vi "FPGA-7842R-Control V1.vi"(0 "Waveform Data":T4, 2 "Action":T5=enum."Exit", 5 "Laser Controls":T1 {"405 Power (0-5V)" min=0.0 max=5.0}, 7 "Manual Controls":T3={"Galvo 1 Position (I16)"=-280, "Galvo 2 Position (I16)"=-280, "X Axis Voltage (I16)"=0, "Y Axis Voltage (I16)"=0, "Z Axis Voltage (I16)"=0, "Res Mirror Amp (I16)"=0, "Res Mirror Mute"=FALSE}, 9 "Image Acquisition Parameters":T2={"Scan Type"=enum."Sample Scanning", "Scan Mode"=enum."XY", "Fast Axis Frequency (Hz)"=100.0, "Image Format"=128, "Line Accumulations"=1, "Frames Per Capture"=1, "Frames Accumulations"=1, "Image Dimension (um)"=[], "Number of Z Steps"=1, "Z Steps Size (um)"=1.0, "Pixel Size (nm)"=[]} {"Z Steps Size (um)" min=0.0; "Number of Z Steps" min=1; "Frames Accumulations" min=1; "Frames Per Capture" min=1; "Line Accumulations" min=1; "Image Format" items=["64 x 64"=64, "128 x 128"=128, "256 x 256"=256, "512 x 512"=512, "1024 x 1024"=1024, "2048 x 2048"=2048]}, 11 "Initialize":bool, 12 "Unused Axis Offset (I16)":i16) -> (15 "Initalized":bool)   [LabVIEW 2016]
uses:
  <vilib>/rvi/interface/nirviOpenFPGA/nirviOpenFPGA.xnode
  <vilib>/rvi/interface/nirviMethod/nirviMethod.xnode
  <vilib>/rvi/interface/nirviReadWriteControl/nirviReadWriteControl.xnode
  <vilib>/rvi/interface/nirviCloseFPGA/nirviCloseFPGA.xnode
  FPGA Bitfiles/MainSTEDFPGAProj_FPGATarget_WaveformandLaser_XaHwHstXqlY.lvbitx
  FPGA Target VIs/FPGA-7841R/Waveform and Laser Controls V6.vi
  <vilib>/FPGAPlugInAG/PCIe-7841R/niLvFpga_Open_PCIe-7841R.vi
  FPGA Target VIs/FPGA-7841R/Waveform Scan Parameters.ctl
  NiFpgaLv.dll
  <vilib>/Utility/error.llb/Error Cluster From Error Code.vi
  <vilib>/rvi/errors/niLvFpgaAdjustHostInterfaceError.vi
  <vilib>/FPGAPlugInAG/PCIe-7841R/niLvFpga_Run_PCIe-7841R.vi
  <vilib>/FPGAPlugInAG/PCIe-7841R/niLvFpga_Close_PCIe-7841R.vi
  Waveform Data.ctl
  FPGA-7842R-Reference.ctl
  Manual Controls V2.ctl
  Type Defs/Image Acquisition Parameters.ctl
  Laser Controls.ctl
panel:
  in  "Laser State 02":bool[](array[boolean])=[FALSE, FALSE, TRUE, FALSE, FALSE, FALSE, FALSE, FALSE]
  in  "Laser State 01":bool[](array[boolean])=[FALSE, TRUE, FALSE, FALSE, FALSE, FALSE, FALSE, FALSE]
  in  "Two Color Line by Line":bool
  in  "Laser On Time (Ticks)":u8=25
  in  "Laser Delay (Ticks)":u8=25
  # "XY"
  # "Z"
  # "Length"
  # "Height"
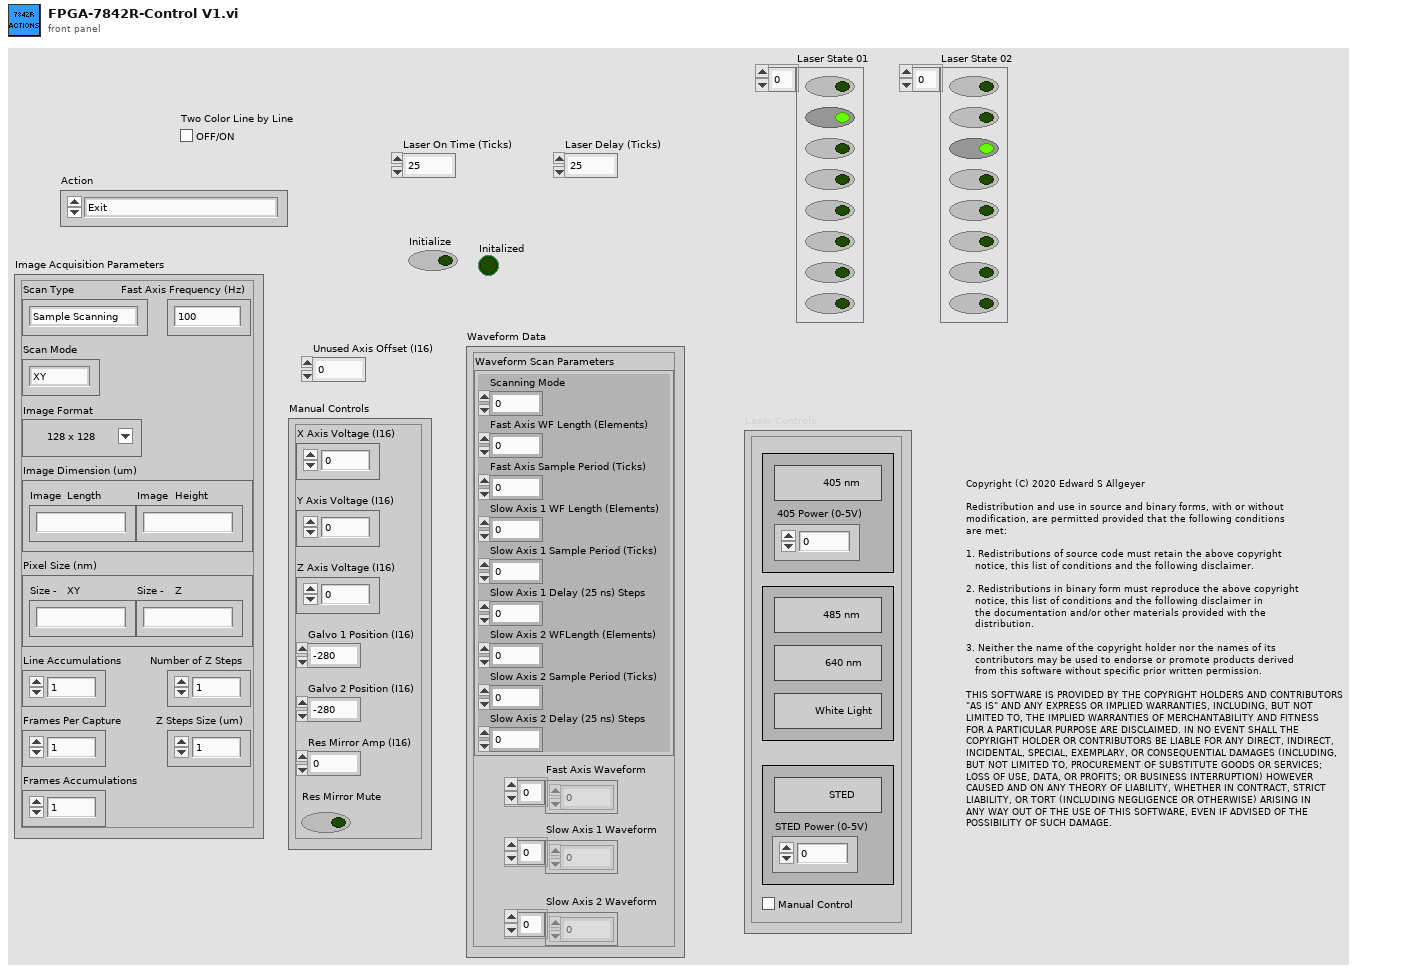
[diagram p1: front panel]
types:
  T1 = typedef "Laser Controls.ctl" = cluster{"STED Power (0-5V)":dbl, "STED":bool, "640 nm":bool, "485 nm":bool, "Manual Control":bool, "White Light":bool, "405 nm":bool, "405 Power (0-5V)":dbl}
  T2 = typedef "Image Acquisition Parameters.ctl" = cluster{"Scan Type":enum16{"Sample Scanning", "Beam Scanning"}, "Scan Mode":enum16{"XY", "XZ", "YZ", "XYZ"}, "Fast Axis Frequency (Hz)":dbl, "Image Format":u16, "Line Accumulations":u16, "Frames Per Capture":u16, "Frames Accumulations":u16, "Image Dimension (um)":dbl[], "Number of Z Steps":u8, "Z Steps Size (um)":dbl, "Pixel Size (nm)":dbl[]}
  T3 = typedef "Manual Controls V2.ctl" = cluster{"Galvo 1 Position (I16)":i16, "Galvo 2 Position (I16)":i16, "X Axis Voltage (I16)":i16, "Y Axis Voltage (I16)":i16, "Z Axis Voltage (I16)":i16, "Res Mirror Amp (I16)":i16, "Res Mirror Mute":bool}
  T4 = typedef "Waveform Data.ctl" = cluster{"Waveform Scan Parameters":cluster{"Scanning Mode":u8, "Fast Axis WF Length (Elements)":i32, "Fast Axis Sample Period (Ticks)":u32, "Slow Axis 1 WF Length (Elements)":i32, "Slow Axis 1 Sample Period (Ticks)":u32, "Slow Axis 1 Delay (25 ns) Steps":i32, "Slow Axis 2 WFLength (Elements)":i32, "Slow Axis 2 Sample Period (Ticks)":u32, "Slow Axis 2 Delay (25 ns) Steps":i32}, "Fast Axis Waveform":dbl[], "Slow Axis 1 Waveform":dbl[], "Slow Axis 2 Waveform":dbl[]}
  T5 = typedef "FPGA-7842R-Reference.ctl" = enum16{"Stage Control", "Laser Control", "Unused Axis I16", "Exit", "Set Res Mirror", "Set Galvo", "Default", "Close FPGA", "Stop Waveforms", "Start Waveforms", "Initialize"}
  T6 = cluster{"Scanning Mode":u8, "Fast Axis WF Length (Elements)":i32, "Fast Axis Sample Period (Ticks)":u32, "Slow Axis 1 WF Length (Elements)":i32, "Slow Axis 1 Sample Period (Ticks)":u32, "Slow Axis 1 Delay (25 ns) Steps":i32, "Slow Axis 2 WFLength (Elements)":i32, "Slow Axis 2 Sample Period (Ticks)":u32, "Slow Axis 2 Delay (25 ns) Steps":i32}
  T7 = cluster{"Res Mirror Amp (I16)":i16, "Res Mirror Mute":bool}
  T8 = typedef "Scan Parameters.ctl" = cluster{"Fast_Ax_Amp_V":dbl, "Fast_Ax_Off_V":dbl, "Slow_Ax_Amp_V":dbl, "Slow_Ax_Off_V ":dbl, "Slow_Ax_Max_V_VperS":dbl, "Slow_Ax1_Del25ns":i32, "Slow_Ax2_Del25ns":i32, "Stage_X_Off_V":dbl, "Stage_Y_Off_V":dbl, "Stage_Z_Off_V":dbl, "Galvo1_Off_V":dbl, "Galvo2_Off_V":dbl, "Last_Scan_Mode":enum16{"XY", "XZ", "YZ", "XYZ"}, "Current_Scan_Mode":enum16{"XY", "XZ", "YZ", "XYZ"}, "Fly_Back_Lines":u16, "Linear_Ramp_End":u32, "Z_Step_I16":i16, "Z_Start_I16":i16, "Laser_States _U32":u32, "590_Voltage_I16":i16, "775_AOM_Volt_I16":i16, "Blanking OFF":bool, "Unused_Axis_I16":i16}
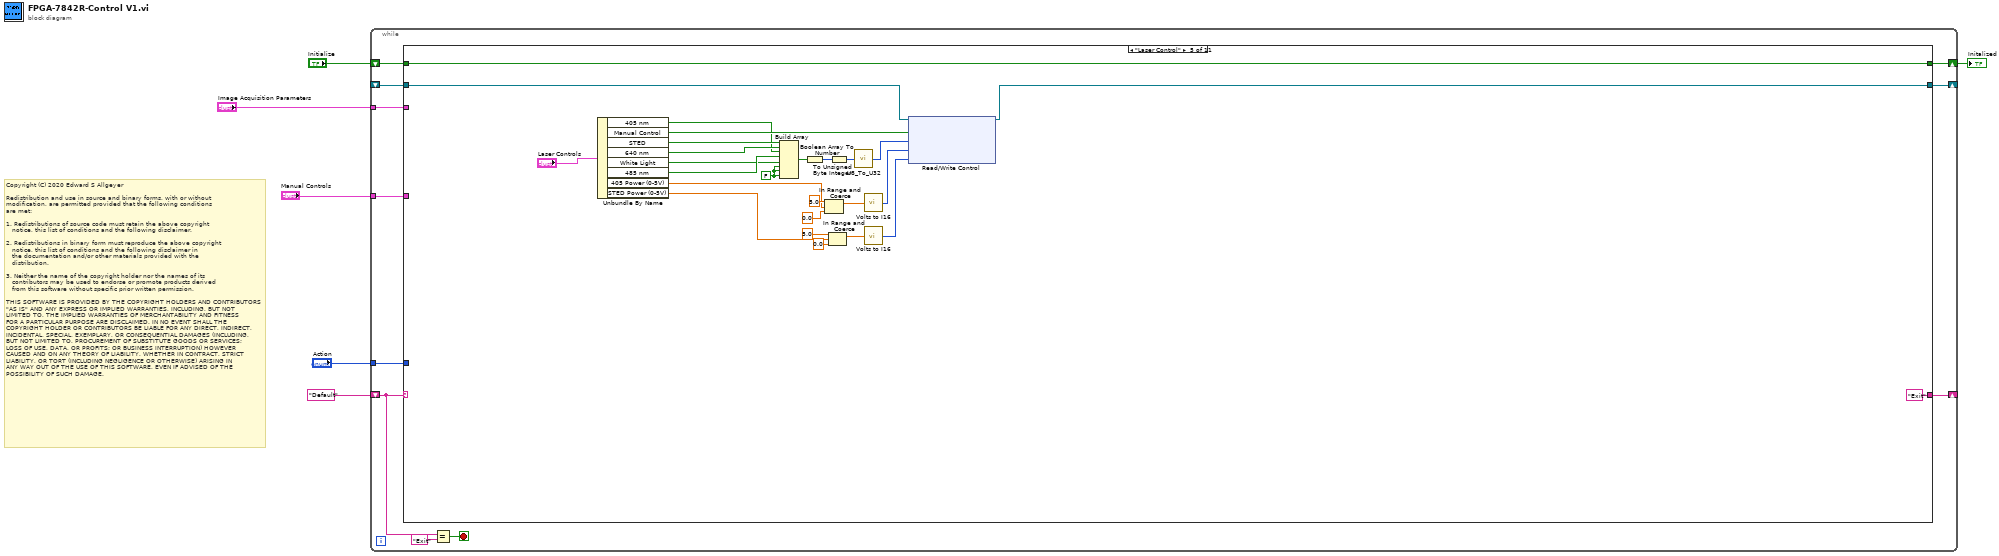
[diagram p0: block diagram]
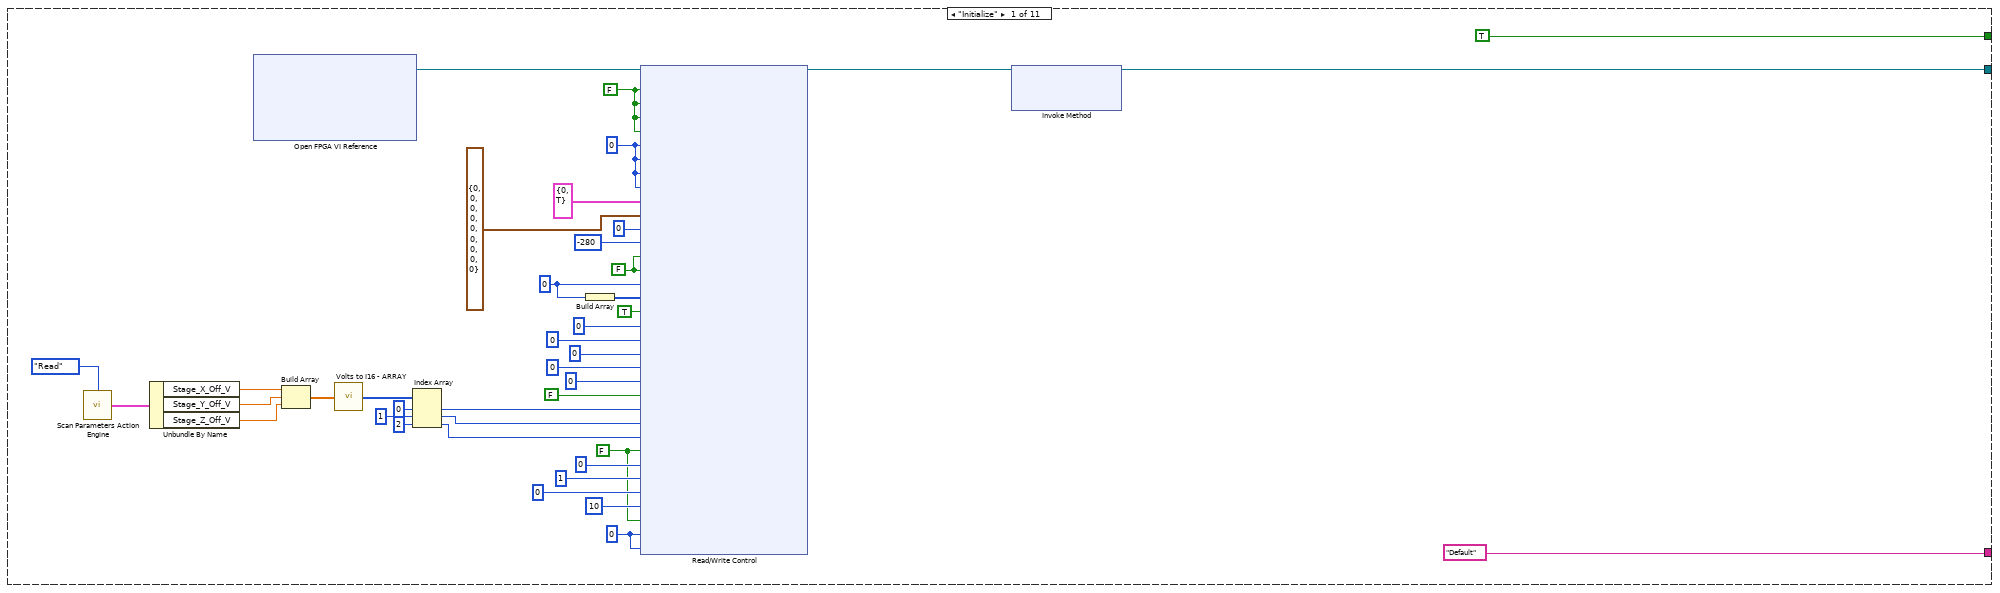
[diagram p2: hidden frame]
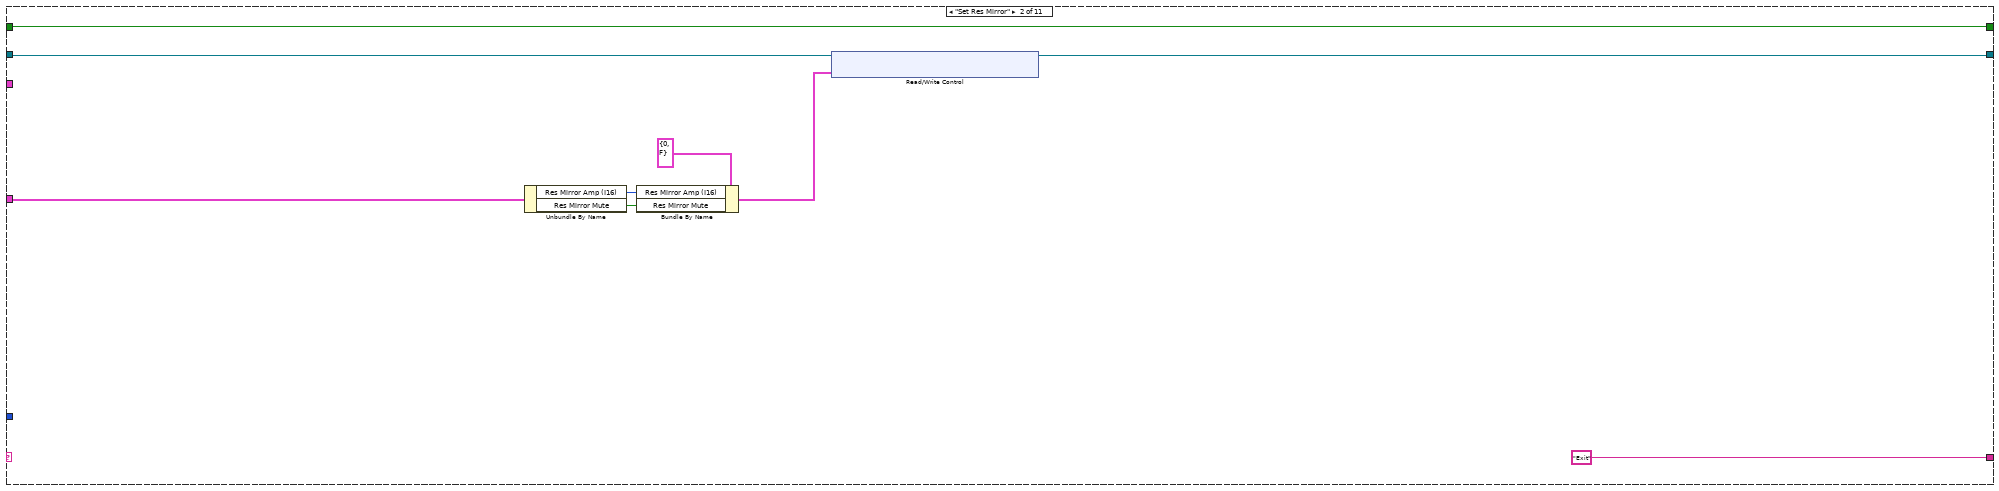
[diagram p3: hidden frame]
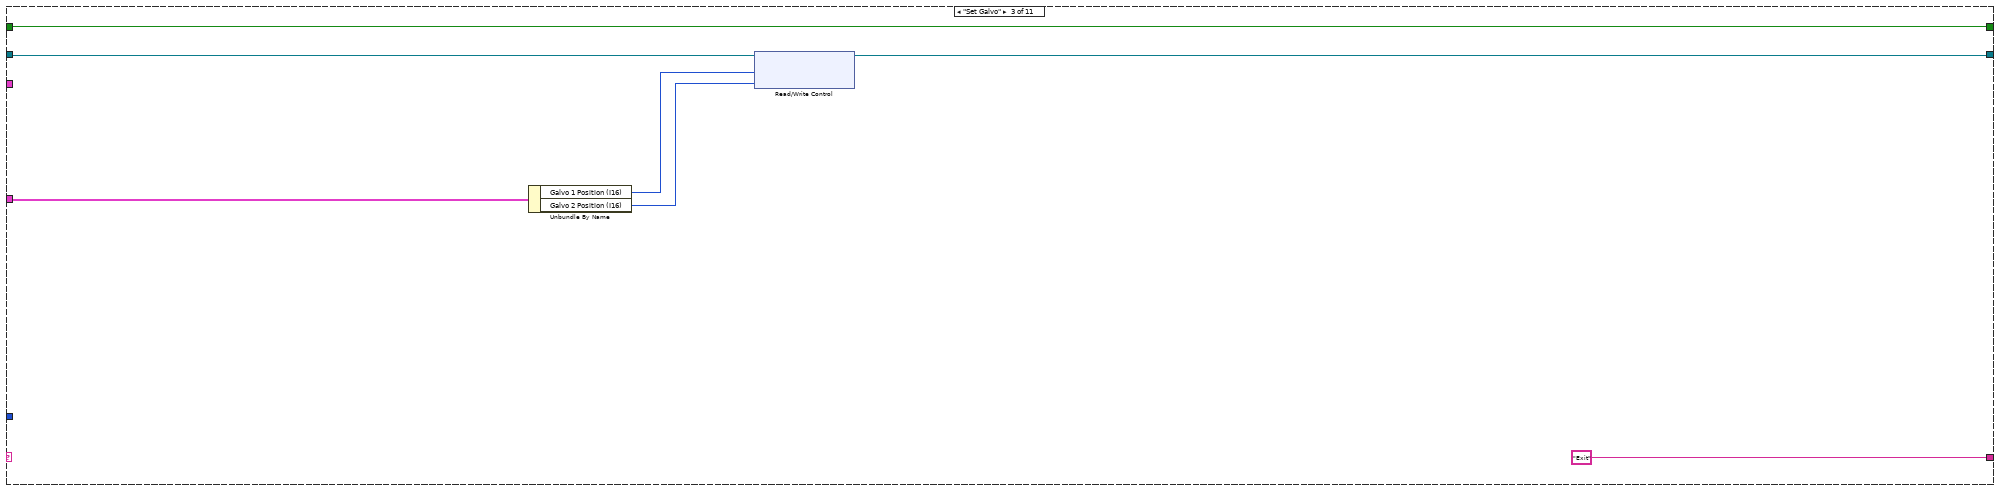
[diagram p4: hidden frame]
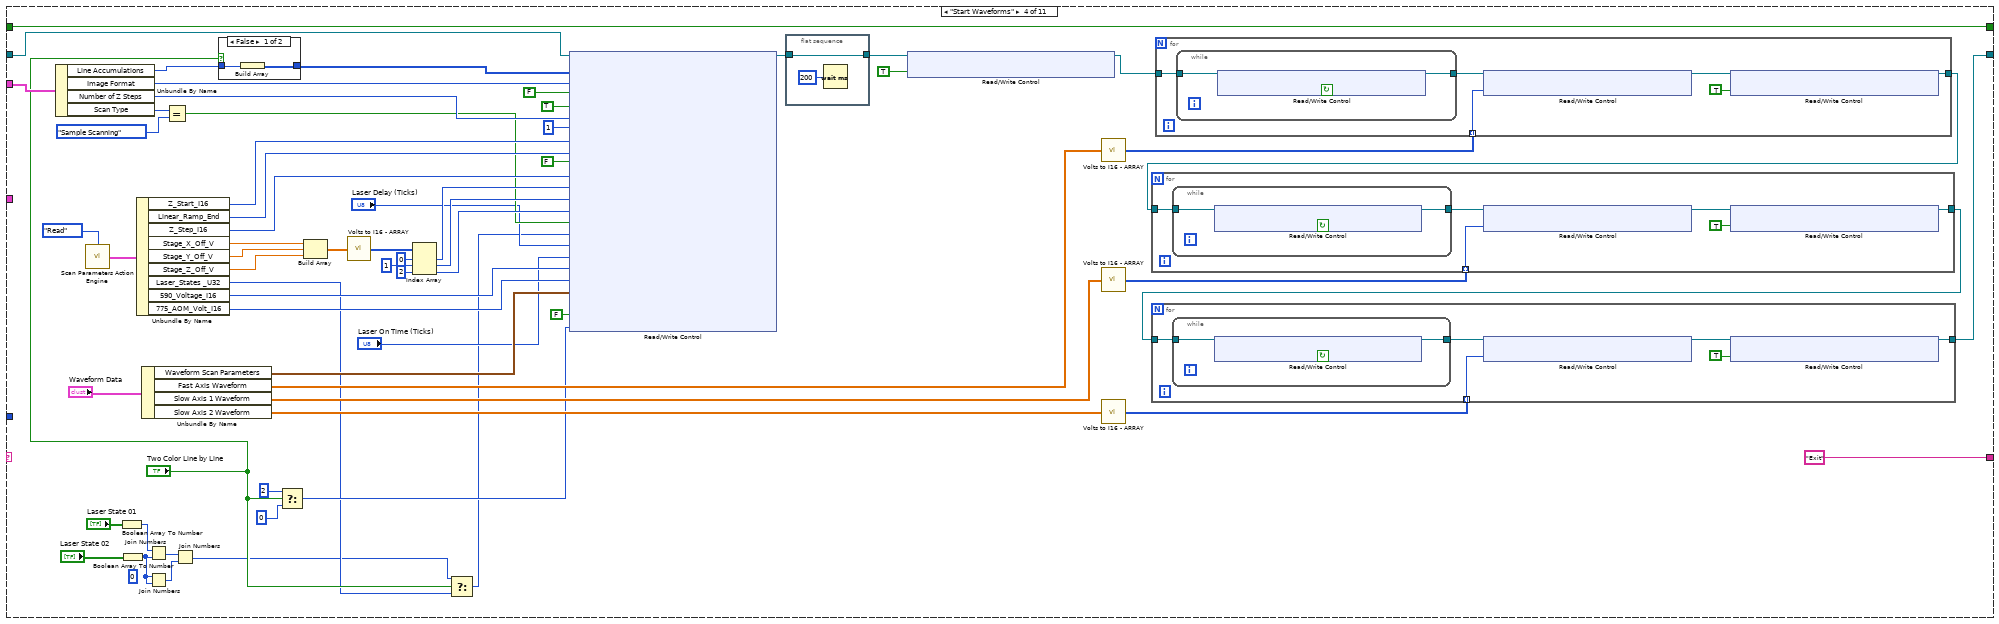
[diagram p5: hidden frame]
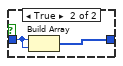
[diagram p6: hidden frame]
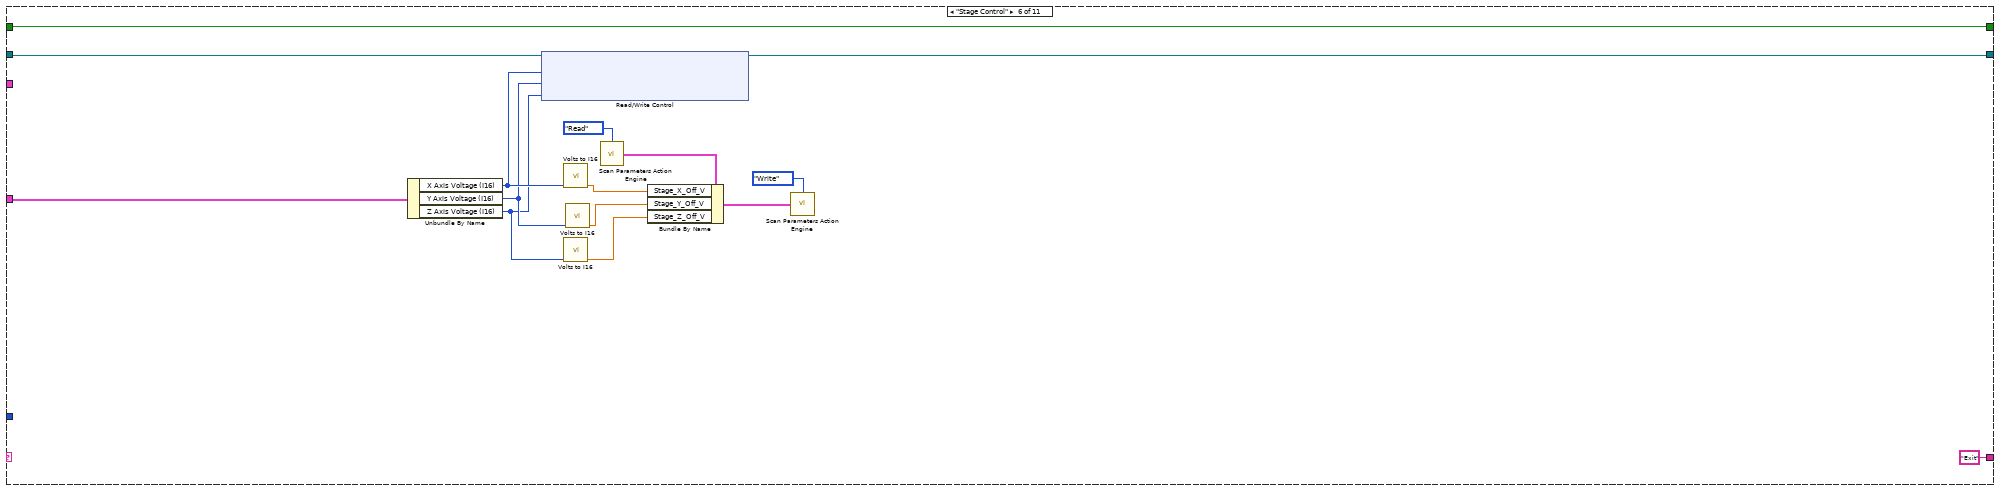
[diagram p7: hidden frame]
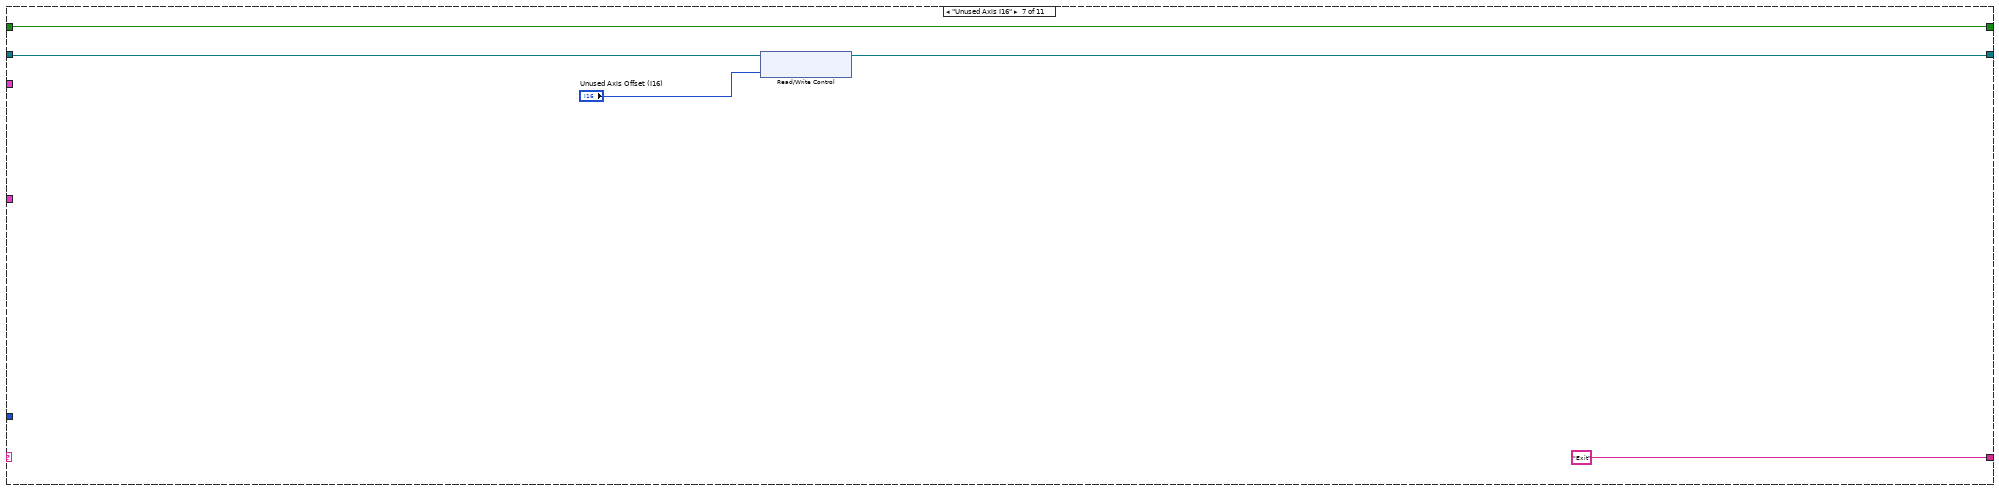
[diagram p8: hidden frame]
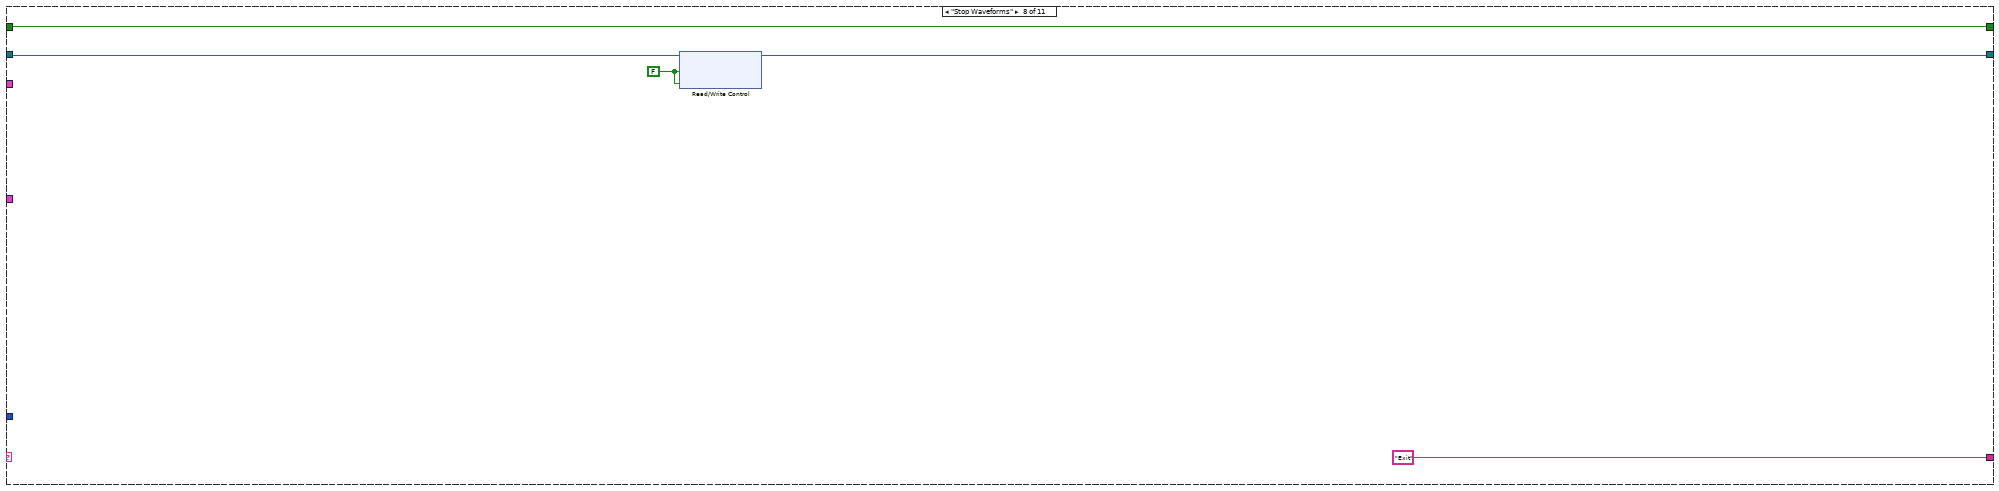
[diagram p9: hidden frame]
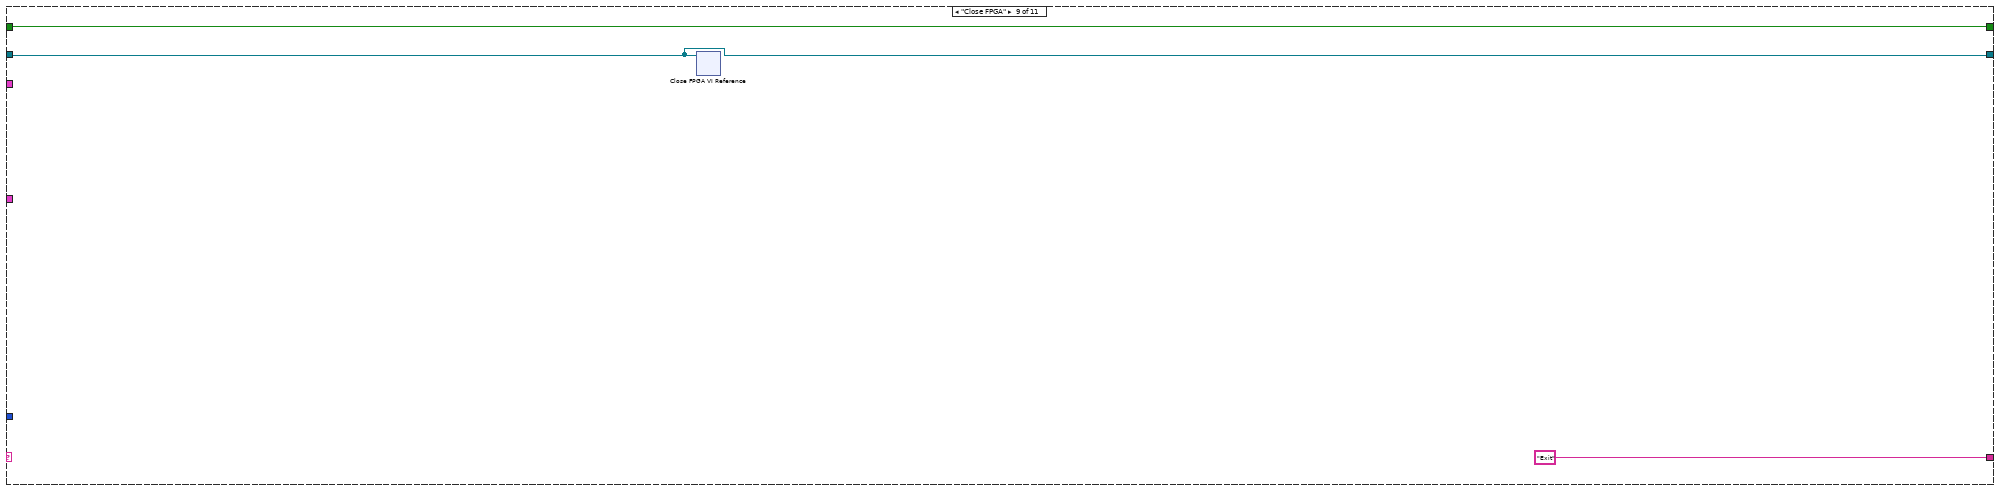
[diagram p10: hidden frame]
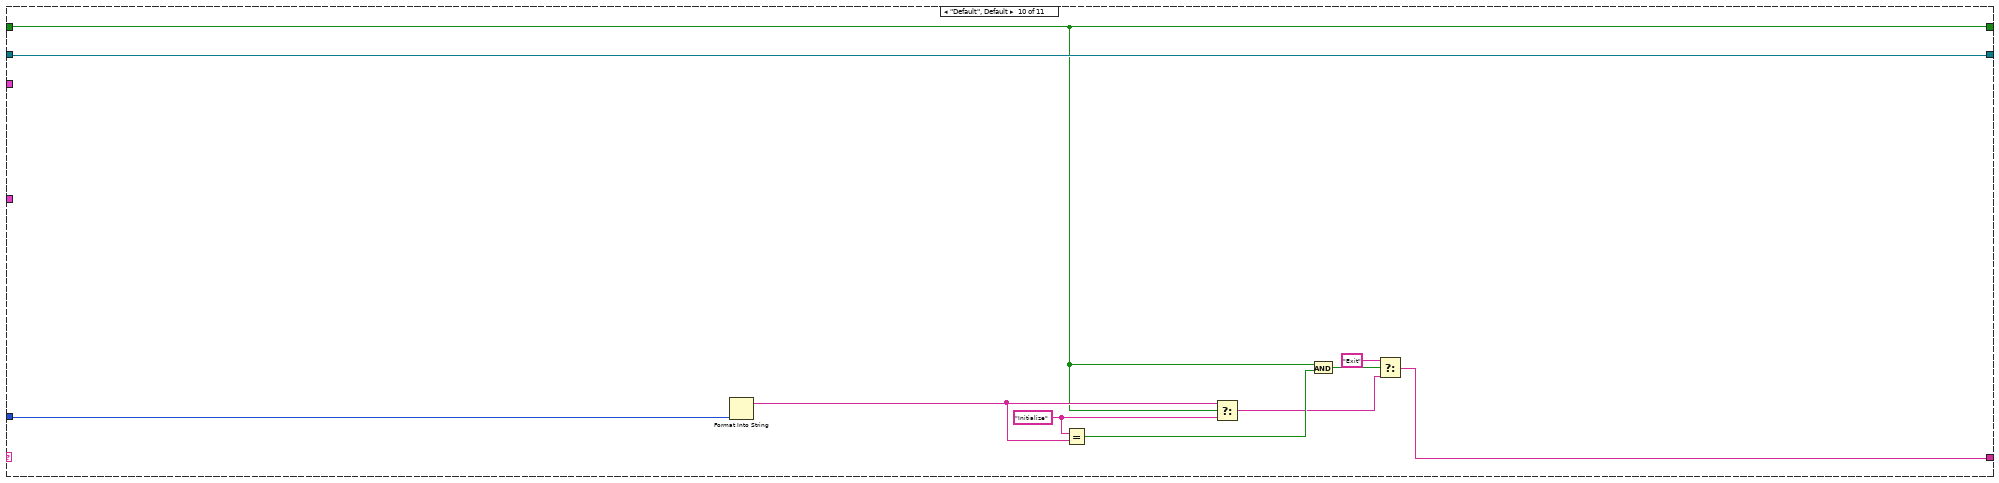
[diagram p11: hidden frame]
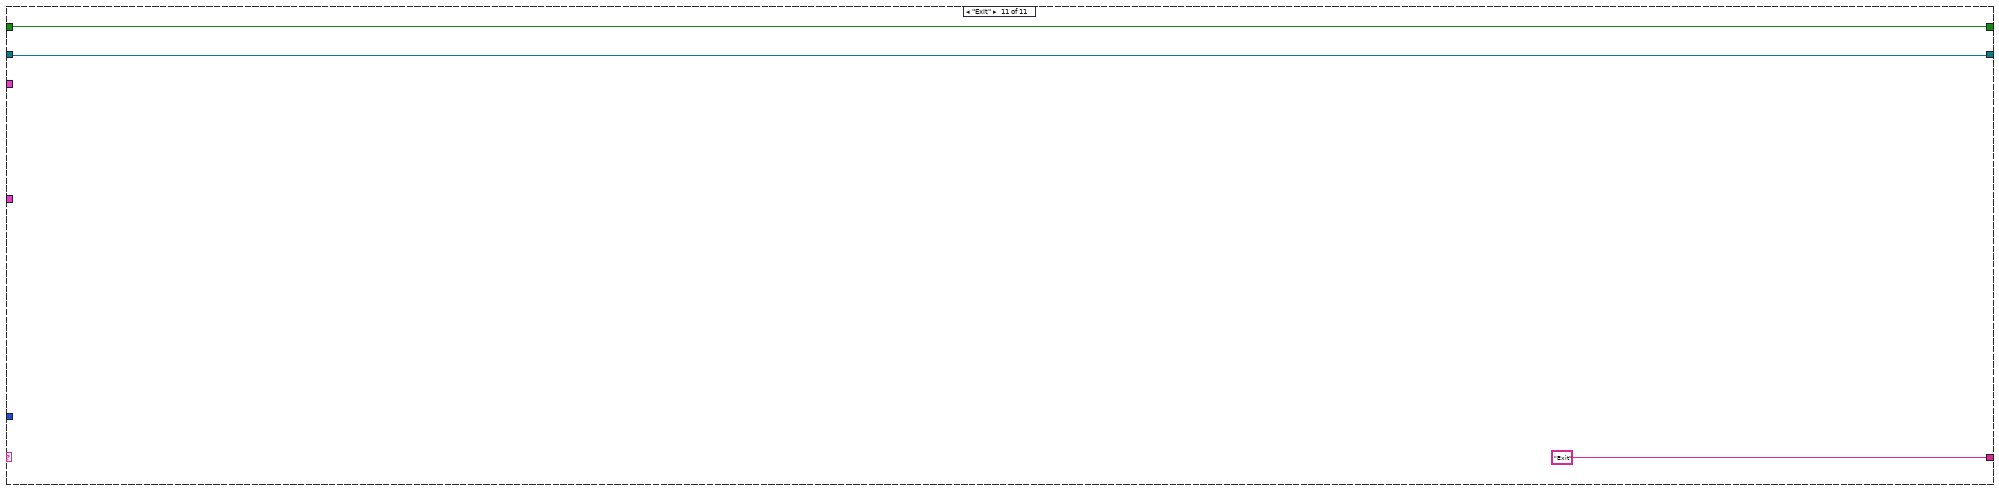
[diagram p12: hidden frame]
diagram:
  # "Copyright (C) 2020 Edward S Allgeyer\n\nRedistribution and use in source and binary forms, with or without\nmodification, are permitted provided that the following conditions\nare met:\n\n1. Redistributions of source code must retain the above copyright\n   notice, this list of conditions and the following disclaimer.\n\n2. Redistributions in binary form must reproduce the above copyright\n   notice, this list of conditions and the following disclaimer in\n   the documentation and/or other materials provided with the\n   distribution.\n\n3. Neither the name of the copyright holder nor the names of its\n   contributors may be used to endorse or promote products derived\n   from this software without specific prior written permission.\n\nTHIS SOFTWARE IS PROVIDED BY THE COPYRIGHT HOLDERS AND CONTRIBUTORS\n\"AS IS\" AND ANY EXPRESS OR IMPLIED WARRANTIES, INCLUDING, BUT NOT\nLIMITED TO, THE IMPLIED WARRANTIES OF MERCHANTABILITY AND FITNESS\nFOR A PARTICULAR PURPOSE ARE DISCLAIMED. IN NO EVENT SHALL THE\nCOPYRIGHT HOLDER OR CONTRIBUTORS BE LIABLE FOR ANY DIRECT, INDIRECT,\nINCIDENTAL, SPECIAL, EXEMPLARY, OR CONSEQUENTIAL DAMAGES (INCLUDING,\nBUT NOT LIMITED TO, PROCUREMENT OF SUBSTITUTE GOODS OR SERVICES;\nLOSS OF USE, DATA, OR PROFITS; OR BUSINESS INTERRUPTION) HOWEVER\nCAUSED AND ON ANY THEORY OF LIABILITY, WHETHER IN CONTRACT, STRICT\nLIABILITY, OR TORT (INCLUDING NEGLIGENCE OR OTHERWISE) ARISING IN\nANY WAY OUT OF THE USE OF THIS SOFTWARE, EVEN IF ADVISED OF THE\nPOSSIBILITY OF SUCH DAMAGE."
  n1 = while {
    shift-right: [w17] -> _
    shift-left: _ -> [w16]
    shift-right: [w14] -> _
    shift-left: "Default" -> [w13]
    tunnel: "Action" -> [w15]
    shift-right: [w10] -> w3
    shift-left: "Initialize" -> [w9]
    tunnel: "Manual Controls" -> [w8]
    tunnel: "Image Acquisition Parameters" -> [w7]
    stop <- w11 stop-if-true
    n2 = case shown="\"Laser Control\"" w13 {
      tunnel: [w48 w63 w70 w126 w192 w207 w213 w220 w222 w226 w235] -> w17
      tunnel: w16 -> [_ w64 w71 w129 w193 w208 w214 w221 w222 w226 w235]
      tunnel: w15 -> [_ _ _ _ _ _ _ _ _ w234 _]
      tunnel: ["Default" ("f") "Exit" ("f") "Exit" ("f") "Exit" ("f") "Exit" ("f") "Exit" ("f") "Exit" ("f") "Exit" ("f") "Exit" ("f") w229 "Exit" ("f")] -> w14
      tunnel: [TRUE w66 w73 w131 w195 w210 w216 w219 w224 w225 w237] -> w10
      tunnel: w9 -> [_ w66 w73 w131 w195 w210 w216 w219 w224 w225 w237]
      tunnel: w8 -> [_ w62 w69 _ _ w209 _ _ _ _ _]
      tunnel: w7 -> [_ _ _ w120 _ _ _ _ _ _ _]
      frame "Initialize" {
        w18 = i16 0 ("590 Analog Voltage (I16)")
        w19 = FALSE ("Blanking Off/Manual")
        w44 = u16 0 ("Number of Lines")
        w46 = FALSE ("Reset Position Error")
        w57 = i16 0 ("Fast Axis Waveform Element")
        w56 = FALSE ("WF 1 Data Loaded")
        n3 = call "Scan Parameters Action Engine.vi"("Action"=enum16{"Read", "Write"}."Read") -> ("Scan Parameters OUT"=w35:T8)  [unwired: 14 in]
        n4 = Unbundle By Name(w35) -> ("Stage_X_Off_V"=w34:dbl, "Stage_Y_Off_V"=w32:dbl, "Stage_Z_Off_V"=w33:dbl)
        n5 = xnode "Open FPGA VI Reference"() -> ("FPGA VI Reference Out"=w47:refnum<k20>)  [unwired: 2 in, 1 out]
        n6 = Build Array(w34, w32, w33) -> (w31:dbl[])
        n7 = call "Volts to I16 - ARRAY.vi"("Voltage (V)"=w31) -> ("I16"=w30:i16[])  [unwired: 14 in]
        n8 = Index Array(array=w30, index #1=0 ("index"), index #2=1 ("index"), index #3=2 ("index")) -> (element #1=w26:i16, element #2=w24:i16, element #3=w25:i16)
        n9 = Build Array(w44) -> (w43:u16[])
        n10 = xnode "Read/Write Control"("FPGA VI Reference In"=w47, "WF 1 Data Loaded"=w56, "WF 2 Data Loaded"=w56, "WF 3 Data Loaded"=w56, "Start Waveforms"=w56, "Fast Axis Waveform Element"=w57, "Slow Axis 1 Waveform Element"=w57, "Slow Axis 2 Waveform Element"=w57, "Unused Axis Offset"=w57, "Resonant Mirror"=T7 {"Res Mirror Amp (I16)"=0, "Res Mirror Mute"=TRUE} ("Resoance Mirror"), "Waveform Scan Parameters"=T6 {"Scanning Mode"=0, "Fast Axis WF Length (Elements)"=0, "Fast Axis Sample Period (Ticks)"=0, "Slow Axis 1 WF Length (Elements)"=0, "Slow Axis 1 Sample Period (Ticks)"=0, "Slow Axis 1 Delay (25 ns) Steps"=0, "Slow Axis 2 WFLength (Elements)"=0, "Slow Axis 2 Sample Period (Ticks)"=0, "Slow Axis 2 Delay (25 ns) Steps"=0}, "Galvo 2 Position (I16)"=i16 0, "Galvo 1 Position (I16)"=i16 -280, "Reset Position Error"=w46, "Frame Trigger"=w46, "Number of Lines"=w44, "Accums Per Line"=w43, "Stop Sync Signal"=TRUE, "Z Step Size (I16)"=i16 0, "Number of Z Steps"=u8 0, "Frames Per Z Step"=u8 0, "Z Stack Start Position (I16)"=i16 0, "End of Linear Ramp"=u32 0, "End Linear Ramp"=FALSE, "X Piezo Axis"=w26, "Y Piezo Axis"=w24, "Z Piezo Axis"=w25, "Blanking Off/Manual"=w19, "Laser States"=u32 0, "Laser Delay (Ticks)"=u8 1, "Sequences"=u8 0, "Laser On Time (Ticks)"=u8 10, "Laser Blank Trigger"=w19, "590 Analog Voltage (I16)"=w18, "775 AOM (I16)"=w18) -> ("FPGA VI Reference Out"=w53:refnum<k20>)  [unwired: 1 in, 1 out]
        n11 = xnode "Invoke Method"("FPGA VI Reference In"=w53) -> ("FPGA VI Reference Out"=w48:refnum<k20>)  [unwired: 2 in, 1 out]
      }
      frame "Set Res Mirror" {
        n12 = Unbundle By Name(w62) -> ("Res Mirror Amp (I16)"=w61:i16, "Res Mirror Mute"=w60:bool)
        n13 = Bundle By Name(cluster=T7 {"Res Mirror Amp (I16)"=0, "Res Mirror Mute"=FALSE} ("Resoance Mirror"), "Res Mirror Amp (I16)"=w61, "Res Mirror Mute"=w60) -> (w58:T7)
        n14 = xnode "Read/Write Control"("FPGA VI Reference In"=w64, "Resonant Mirror"=w58) -> ("FPGA VI Reference Out"=w63:refnum<k20>)  [unwired: 1 in, 1 out]
      }
      frame "Set Galvo" {
        n15 = Unbundle By Name(w69) -> ("Galvo 1 Position (I16)"=w68:i16, "Galvo 2 Position (I16)"=w67:i16)
        n16 = xnode "Read/Write Control"("FPGA VI Reference In"=w71, "Galvo 1 Position (I16)"=w68, "Galvo 2 Position (I16)"=w67) -> ("FPGA VI Reference Out"=w70:refnum<k20>)  [unwired: 1 in, 1 out]
      }
      frame "Start Waveforms" {
        (unwired) u8 0
        n17 = Unbundle By Name(w120) -> ("Line Accumulations"=w118:u16, "Image Format"=w119:u16, "Number of Z Steps"=w109:u8, "Scan Type"=w95:enum16{"Sample Scanning", "Beam Scanning"})
        n18 = call "Scan Parameters Action Engine.vi"("Action"=enum16{"Read", "Write"}."Read") -> ("Scan Parameters OUT"=w113:T8)  [unwired: 14 in]
        n19 = Boolean Array To Number(Boolean array="Laser State 01") -> (number=w78:u8)
        n20 = Boolean Array To Number(Boolean array="Laser State 02") -> (number=w74:u8)
        n21 = Unbundle By Name(w113) -> ("Z_Start_I16"=w111:i16, "Linear_Ramp_End"=w112:u32, "Z_Step_I16"=w108:i16, "Stage_X_Off_V"=w101:dbl, "Stage_Y_Off_V"=w100:dbl, "Stage_Z_Off_V"=w99:dbl, "Laser_States _U32"=w82:u32, "590_Voltage_I16"=w92:i16, "775_AOM_Volt_I16"=w91:i16)
        n22 = Unbundle By Name("Waveform Data") -> ("Waveform Scan Parameters"=w90:T6, "Fast Axis Waveform"=w133:dbl[], "Slow Axis 1 Waveform"=w125:dbl[], "Slow Axis 2 Waveform"=w132:dbl[])
        n23 = Join Numbers(hi=w78, lo=w74) -> ((hi.lo)=w79:u16)
        n24 = Join Numbers(hi=w74, lo=w74) -> ((hi.lo)=w80:u16)
        n25 = Equal?(x=w95, y=enum16{"Sample Scanning", "Beam Scanning"}."Sample Scanning" ("Scan Type")) -> (x = y?=w93:bool)
        n26 = Join Numbers(hi=w79, lo=w80) -> ((hi.lo)=w75:u32)
        n27 = case shown="False" "Two Color Line by Line" {
          tunnel: w118 -> [w139 w140]
          tunnel: [w138 w141] -> w117
          frame False {
            n28 = Build Array(w139) -> (w138:u16[])
          }
          frame True {
            n29 = Build Array(w140, w140) -> (w141:u16[])
          }
        }
        n30 = Select(t=u8 2, s="Two Color Line by Line", f=u8 0 ("Sequences")) -> (s? t:f=w84:u8)
        n31 = Build Array(w101, w100, w99) -> (w106:dbl[])
        n32 = call "Volts to I16 - ARRAY.vi"("Voltage (V)"=w106) -> ("I16"=w105:i16[])  [unwired: 14 in]
        n33 = Index Array(array=w105, index #1=0 ("index"), index #2=1 ("index"), index #3=2 ("index")) -> (element #1=w98:i16, element #2=w97:i16, element #3=w96:i16)
        n34 = Select(t=w75, s="Two Color Line by Line", f=w82) -> (s? t:f=w81:u32)
        n35 = xnode "Read/Write Control"("FPGA VI Reference In"=w129, "Accums Per Line"=w117, "Number of Lines"=w119, "Frame Trigger"=FALSE, "Stop Sync Signal"=TRUE, "Number of Z Steps"=w109, "Frames Per Z Step"=u8 1, "Z Stack Start Position (I16)"=w111, "End of Linear Ramp"=w112, "End Linear Ramp"=FALSE, "Z Step Size (I16)"=w108, "X Piezo Axis"=w98, "Y Piezo Axis"=w97, "Z Piezo Axis"=w96, "Blanking Off/Manual"=w93, "Laser States"=w81, "Laser Delay (Ticks)"="Laser Delay (Ticks)", "Laser On Time (Ticks)"="Laser On Time (Ticks)", "590 Analog Voltage (I16)"=w92, "775 AOM (I16)"=w91, "Waveform Scan Parameters"=w90, "Frame Trigger"=FALSE, "Sequences"=w84) -> ("FPGA VI Reference Out"=w127:refnum<k20>)  [unwired: 1 in, 2 out]
        n36 = flat-sequence {
          tunnel: [w143] -> w128
          tunnel: w127 -> [w143]
          frame #0 {
            n37 = Wait (ms)(milliseconds to wait=u32 200) -> ()  [unwired: 1 out]
          }
        }
        n38 = xnode "Read/Write Control"("FPGA VI Reference In"=w128, "Start Waveforms"=TRUE) -> ("FPGA VI Reference Out"=w134:refnum<k20>)  [unwired: 1 in, 1 out]
        n39 = call "Volts to I16 - ARRAY.vi"("Voltage (V)"=w133) -> ("I16"=w137:i16[])  [unwired: 14 in]
        n40 = call "Volts to I16 - ARRAY.vi"("Voltage (V)"=w125) -> ("I16"=w123:i16[])  [unwired: 14 in]
        n41 = call "Volts to I16 - ARRAY.vi"("Voltage (V)"=w132) -> ("I16"=w124:i16[])  [unwired: 14 in]
        n42 = for {
          tunnel: w134 -> [w166]
          tunnel: [w164] -> w136
          tunnel: w137 -> [w162] mode=indexing
          n43 = while {
            tunnel: w166 -> [w170]
            tunnel: [w169] -> w165
            stop <- w168 continue-if-true
            n44 = xnode "Read/Write Control"("FPGA VI Reference In"=w170) -> ("FPGA VI Reference Out"=w169:refnum<k20>, "WF 1 Data Loaded"=w168:bool)  [unwired: 1 in, 1 out]
          }
          n45 = xnode "Read/Write Control"("FPGA VI Reference In"=w165, "Fast Axis Waveform Element"=w162) -> ("FPGA VI Reference Out"=w167:refnum<k20>)  [unwired: 1 in, 1 out]
          n46 = xnode "Read/Write Control"("FPGA VI Reference In"=w167, "WF 1 Data Loaded"=TRUE ("Host Data Loaded")) -> ("FPGA VI Reference Out"=w164:refnum<k20>)  [unwired: 1 in, 1 out]
        }
        n47 = for {
          tunnel: w136 -> [w157]
          tunnel: [w155] -> w107
          tunnel: w123 -> [w153] mode=indexing
          n48 = while {
            tunnel: w157 -> [w161]
            tunnel: [w160] -> w156
            stop <- w159 continue-if-true
            n49 = xnode "Read/Write Control"("FPGA VI Reference In"=w161) -> ("FPGA VI Reference Out"=w160:refnum<k20>, "WF 2 Data Loaded"=w159:bool)  [unwired: 1 in, 1 out]
          }
          n50 = xnode "Read/Write Control"("FPGA VI Reference In"=w156, "Slow Axis 1 Waveform Element"=w153) -> ("FPGA VI Reference Out"=w158:refnum<k20>)  [unwired: 1 in, 1 out]
          n51 = xnode "Read/Write Control"("FPGA VI Reference In"=w158, "WF 2 Data Loaded"=TRUE ("Host Data Loaded")) -> ("FPGA VI Reference Out"=w155:refnum<k20>)  [unwired: 1 in, 1 out]
        }
        n52 = for {
          tunnel: w107 -> [w148]
          tunnel: [w146] -> w126
          tunnel: w124 -> [w144] mode=indexing
          n53 = while {
            tunnel: w148 -> [w152]
            tunnel: [w151] -> w147
            stop <- w150 continue-if-true
            n54 = xnode "Read/Write Control"("FPGA VI Reference In"=w152) -> ("FPGA VI Reference Out"=w151:refnum<k20>, "WF 3 Data Loaded"=w150:bool)  [unwired: 1 in, 1 out]
          }
          n55 = xnode "Read/Write Control"("FPGA VI Reference In"=w147, "Slow Axis 2 Waveform Element"=w144) -> ("FPGA VI Reference Out"=w149:refnum<k20>)  [unwired: 1 in, 1 out]
          n56 = xnode "Read/Write Control"("FPGA VI Reference In"=w149, "WF 3 Data Loaded"=TRUE ("Host Data Loaded")) -> ("FPGA VI Reference Out"=w146:refnum<k20>)  [unwired: 1 in, 1 out]
        }
      }
      frame "Laser Control" {
        w184 = FALSE ("element")
        n57 = Unbundle By Name("Laser Controls") -> ("405 nm"=w173:bool, "Manual Control"=w194:bool, "STED"=w181:bool, "640 nm"=w180:bool, "White Light"=w174:bool, "485 nm"=w179:bool, "405 Power (0-5V)"=w171:dbl, "STED Power (0-5V)"=w172:dbl)
        n58 = Build Array(w181, w180, w173, w179, w174, w184, w184, w184) -> (w182:bool[])
        n59 = Boolean Array To Number(Boolean array=w182) -> (number=w183:u32)
        n60 = In Range and Coerce(upper limit=5.0, x=w171, lower limit=0.0) -> (coerced(x)=w189:dbl)  [unwired: 1 out]
        n61 = In Range and Coerce(upper limit=5.0, x=w172, lower limit=0.0) -> (coerced(x)=w190:dbl)  [unwired: 1 out]
        n62 = To Unsigned Byte Integer(number=w183) -> (unsigned 8bit integer=w185:u8)
        n63 = call "U8_To_U32.vi"("U8 IN"=w185) -> ("U32 OUT"=w178:u32)  [unwired: 13 in, 1 out]
        n64 = call "Volts to I16.vi"("Voltage (V)"=w189) -> ("I16"=w177:i16)  [unwired: 13 in, 1 out]
        n65 = call "Volts to I16.vi"("Voltage (V)"=w190) -> ("I16"=w176:i16)  [unwired: 13 in, 1 out]
        n66 = xnode "Read/Write Control"("FPGA VI Reference In"=w193, "Blanking Off/Manual"=w194, "Laser States"=w178, "590 Analog Voltage (I16)"=w177, "775 AOM (I16)"=w176) -> ("FPGA VI Reference Out"=w192:refnum<k20>)  [unwired: 1 in, 1 out]
      }
      frame "Stage Control" {
        n67 = Unbundle By Name(w209) -> ("X Axis Voltage (I16)"=w204:i16, "Y Axis Voltage (I16)"=w200:i16, "Z Axis Voltage (I16)"=w199:i16)
        n68 = xnode "Read/Write Control"("FPGA VI Reference In"=w208, "X Piezo Axis"=w204, "Y Piezo Axis"=w200, "Z Piezo Axis"=w199) -> ("FPGA VI Reference Out"=w207:refnum<k20>)  [unwired: 1 in, 1 out]
        n69 = call "Volts to I16.vi"("Volatge (I16)"=w204) -> ("Voltage (V)"=w203:dbl)  [unwired: 13 in, 1 out]
        n70 = call "Volts to I16.vi"("Volatge (I16)"=w199) -> ("Voltage (V)"=w201:dbl)  [unwired: 13 in, 1 out]
        n71 = call "Volts to I16.vi"("Volatge (I16)"=w200) -> ("Voltage (V)"=w202:dbl)  [unwired: 13 in, 1 out]
        n72 = call "Scan Parameters Action Engine.vi"("Action"=enum16{"Read", "Write"}."Read") -> ("Scan Parameters OUT"=w205:T8)  [unwired: 14 in]
        n73 = Bundle By Name(cluster=w205, "Stage_X_Off_V"=w203, "Stage_Y_Off_V"=w202, "Stage_Z_Off_V"=w201) -> (w197:T8)
        n74 = call "Scan Parameters Action Engine.vi"("Action"=enum16{"Read", "Write"}."Write", "Scan Parameters IN"=w197) -> ()  [unwired: 13 in, 1 out]
      }
      frame "Unused Axis I16" {
        n75 = xnode "Read/Write Control"("FPGA VI Reference In"=w214, "Unused Axis Offset"="Unused Axis Offset (I16)") -> ("FPGA VI Reference Out"=w213:refnum<k20>)  [unwired: 1 in, 1 out]
      }
      frame "Stop Waveforms" {
        w217 = FALSE ("Start Waveforms")
        n76 = xnode "Read/Write Control"("FPGA VI Reference In"=w221, "Start Waveforms"=w217, "Stop Sync Signal"=w217) -> ("FPGA VI Reference Out"=w220:refnum<k20>)  [unwired: 1 in, 1 out]
      }
      frame "Close FPGA" {
        n77 = xnode "Close FPGA VI Reference"("FPGA VI Reference In"=w222) -> ()  [unwired: 1 in, 1 out]
      }
      frame "Default", Default {
        w228 = "Initialize" ("f")
        n78 = Format Into String(w234) -> (resulting string=w227:string)  [unwired: 3 in, 1 out]
        n79 = Equal?(x=w228, y=w227) -> (x = y?=w233:bool)
        n80 = Select(t=w227, s=w225, f=w228) -> (s? t:f=w230:string)
        n81 = And(x=w225, y=w233) -> (x .and. y?=w232:bool)
        n82 = Select(t="Exit" ("y"), s=w232, f=w230) -> (s? t:f=w229:string)
      }
      frame "Exit" {
      }
    }
    n83 = Equal?(x=w13, y="Exit") -> (x = y?=w11:bool)
  }
  "Initalized" <- w3
